vi "Cal Constants Cluster to Array.vi"(11 "Cluster":T1) -> (3 "Array":dbl[](array[numeric]))   [LabVIEW 2024]
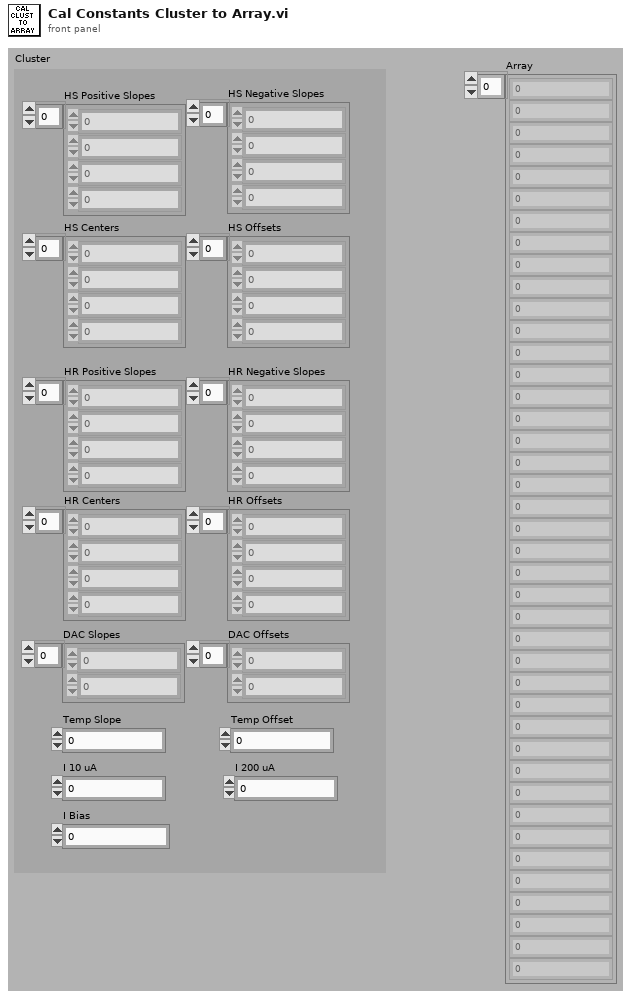
[diagram p1: front panel]
types:
  T1 = cluster{"HS Positive Slopes":dbl[], "HS Negative Slopes":dbl[], "HS Centers":dbl[], "HS Offsets":dbl[], "HR Positive Slopes":dbl[], "HR Negative Slopes":dbl[], "HR Centers":dbl[], "HR Offsets":dbl[], "DAC Slopes":dbl[], "DAC Offsets":dbl[], "Temp Slope":dbl, "Temp Offset":dbl, "I 10 uA":dbl, "I 200 uA":dbl, "I Bias":dbl}
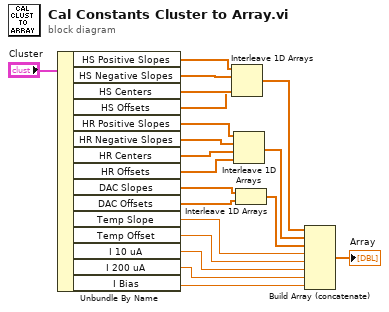
[diagram p0: block diagram]
diagram:
  n1 = Unbundle By Name("Cluster") -> ("HS Positive Slopes"=w19:dbl[], "HS Negative Slopes"=w18:dbl[], "HS Centers"=w17:dbl[], "HS Offsets"=w16:dbl[], "HR Positive Slopes"=w15:dbl[], "HR Negative Slopes"=w14:dbl[], "HR Centers"=w13:dbl[], "HR Offsets"=w12:dbl[], "DAC Slopes"=w11:dbl[], "DAC Offsets"=w10:dbl[], "Temp Slope"=w5:dbl, "Temp Offset"=w6:dbl, "I 10 uA"=w7:dbl, "I 200 uA"=w8:dbl, "I Bias"=w9:dbl)
  n2 = Interleave 1D Arrays(w19, w18, w17, w16) -> (w2:dbl[])
  n3 = Interleave 1D Arrays(w15, w14, w13, w12) -> (w3:dbl[])
  n4 = Interleave 1D Arrays(w11, w10) -> (w4:dbl[])
  n5 = Build Array (concatenate)(w2, w3, w4, w5, w6, w7, w8, w9) -> (→"Array":dbl[])
